vi "WriteConfig.vi"(11 "Path":path=path "/home/lvuser/sirius.conf") -> ()   [LabVIEW 2015]
uses:
  Support/Global Objects.vi
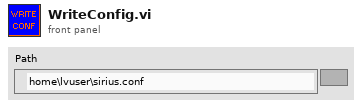
[diagram p1: front panel]
types:
  T1 = typedef "Configuration.ctl" = cluster{"Throttle Dead Zone":dbl, "Throttle Ramp Rate":dbl, "Turn Dead Zone":dbl, "Auton":cluster{"Motion Plan P":dbl, "Motion Plan I":dbl, "Motion Plan D":dbl}, "Auto Upshift Enabled":bool, "Upshift Min Throttle":dbl, "Upshift Min Velocity":dbl, "Min time before upshift":dbl, "Shift Throttle Detent":u32, "Min time before downshift":dbl, "Turn PID":cluster{"Motion Plan P":dbl, "Motion Plan I":dbl, "Motion Plan D":dbl}, "Auto Coast Downshift":bool, "Downshift Coast Max Vel":dbl, "Downshift Coast Throttle Epsilon":dbl, "Left Motor Calibration":dbl, "Right Motor Calibration":dbl, "Tank Mode":bool, "Shooter PID":cluster{"Shooter  P":dbl, "Shooter  I":dbl, "Shooter  D":dbl}}
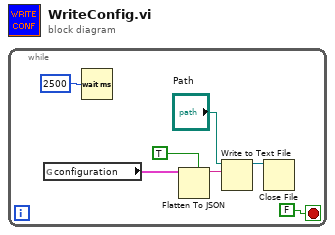
[diagram p0: block diagram]
diagram:
  n1 = while {
    stop <- FALSE stop-if-true
    n2 = global read "Global Objects.vi" "configuration"() -> (w1:T1)
    n3 = Wait (ms)(milliseconds to wait=u32 2500) -> ()  [unwired: 1 out]
    n4 = Flatten To JSON(enable LabVIEW extensions? (T)=TRUE, anything=w1) -> (JSON string=w5:string)  [unwired: 1 in, 1 out]
    n5 = Write to Text File(file (use dialog)="Path", text=w5) -> (refnum out=w3:refnum<file>)  [unwired: 2 in, 2 out]
    n6 = Close File(refnum=w3) -> ()  [unwired: 1 in, 2 out]
  }
